vi "LVClass_Camera ctor.vi"(0 "Camera (const)":refnum<class "Camera.lvclass">, 5 "Configuration file path":path, 11 "error in (no error)":errorcluster) -> (4 "Camera (new)":refnum<class "Camera.lvclass">, 15 "error out":errorcluster)   [LabVIEW 2020, in "Camera.lvclass"]
doc: "Camera constructor.\n\n<B>CameraIn</B> : Constant Pointer to Camera object, Camera connection is automatically\n established to the device. (no neeed to use Imop_Camera_Connect)\n<B>CameraOut</B> : Constant Pointer to Camera object, Camera connection is automatically\n established to the device. (no neeed to use Imop_Camera_Connect)\n<B>config_file_path</B> : Absolute path to Haso or Camera configuration file."
uses:
  Camera.lvclass
  Handle creation.ctl
  Camera.lvclass/Camera.ctl
  CameraSet.lvclass
  Image.lvclass
  Data alignment enum.ctl
  CameraAcquisitionState.ctl
  LVClass_CameraSet Read CameraParameters.vi
  LVClass_CameraSet Read AllValueSetAndGet.vi
  LVClass_CameraSet Read AllValueGet.vi
panel:
  out "Iteration":i32
  out "State":i32
  out "path to wavekit library":path
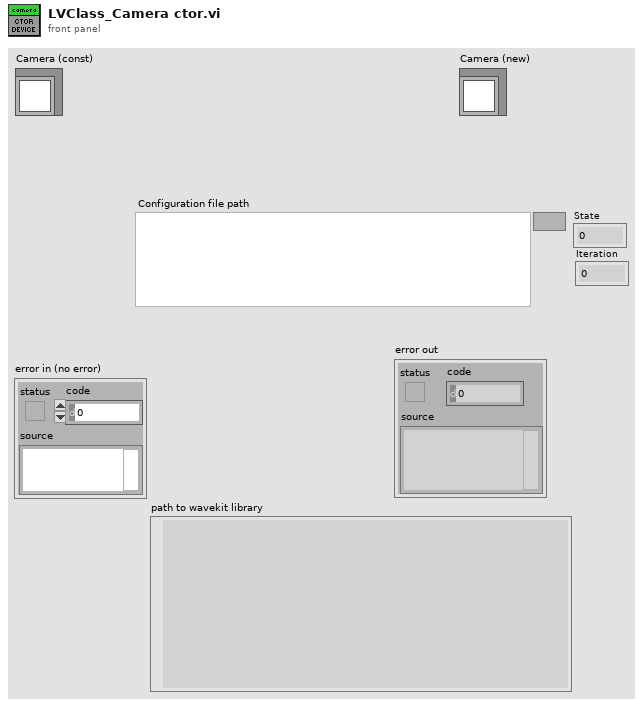
[diagram p1: front panel]
types:
  T1 = typedef "Handle creation.ctl" = enum16{"By ctor", "By write function"}
  T2 = typedef "Data alignment enum.ctl" = enum16{"8", "16", "32"}
  T3 = typedef "CameraAcquisitionState.ctl" = enum16{"Stop", "Live"}
  T4 = typedef "ParameterID.ctl" = cluster{"Name":string, "ConnectionParameter?":bool, "Type":T5, "Authorization":T6, "OnFlyAuthorization":T7, "StringValue":string, "Value":dbl, "Min":dbl, "Max":dbl, "BooleanValue":bool, "StringParameterList":string[]}
  T5 = typedef "CameraParameters_Type.ctl" = enum16{"Integer", "Real", "String", "Boolean"}
  T6 = typedef "CameraParameters_Authorization.ctl" = enum16{"Disable", "Gettable", "Settable - Gettable"}
  T7 = typedef "CameraParameters_OnFlyAuthorization.ctl" = enum16{"None", "Gettable", "Settable", "Settable - Gettable"}
  T8 = typedef "CameraParametersSetup.ctl" = cluster{"Name":string, "Type":T5, "Value":dbl, "BooleanValue":bool, "StringValue":string, "ConnectionParameter":bool}
  T9 = typedef "CameraSpecifications.ctl" = cluster{"Grabber name":string, "Camera name":string, "Camera sn":string, "Pixels_um":T10, "Maximum level":u32, "Data alignment":T2, "Is signed":bool, "Acquisition start":T11, "Acquisition length":T11, "MaxFrameRate_Hz":sgl, "Chip type":enum16{"Progressive scan", "Frame transfert"}}
  T10 = typedef "General dimensions definition.ctl" = cluster{"Size":T11, "Step":T12}
  T11 = typedef "Point2D.ctl" = cluster{"X":u32, "Y":u32}
  T12 = typedef "Point2Df.ctl" = cluster{"X":sgl, "Y":sgl}
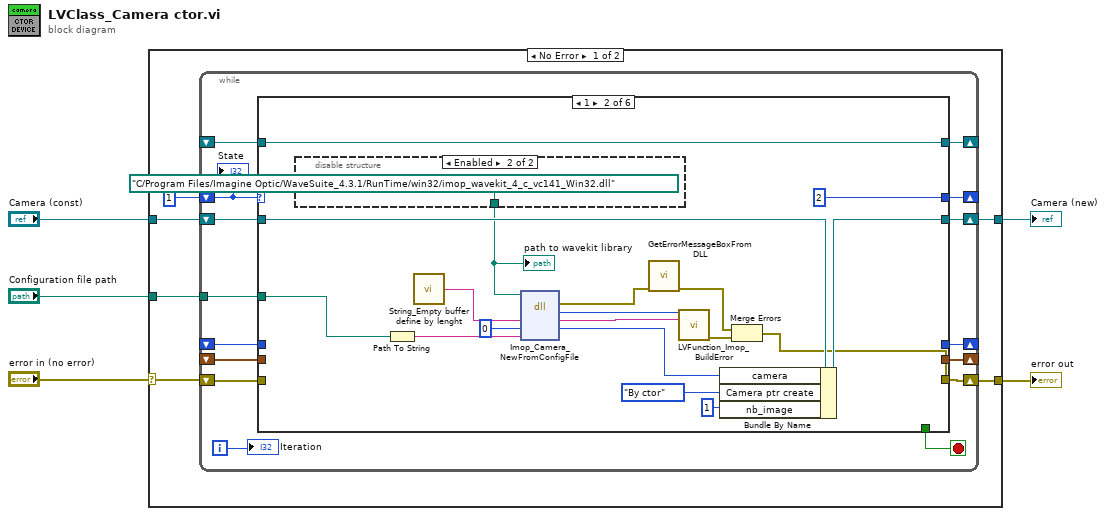
[diagram p0: block diagram]
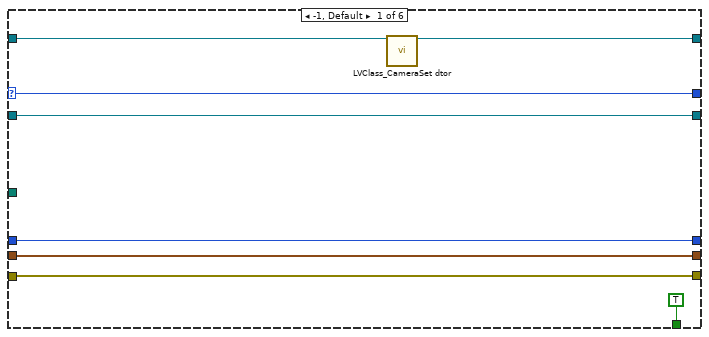
[diagram p2: hidden frame]
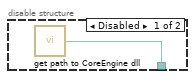
[diagram p3: hidden frame]
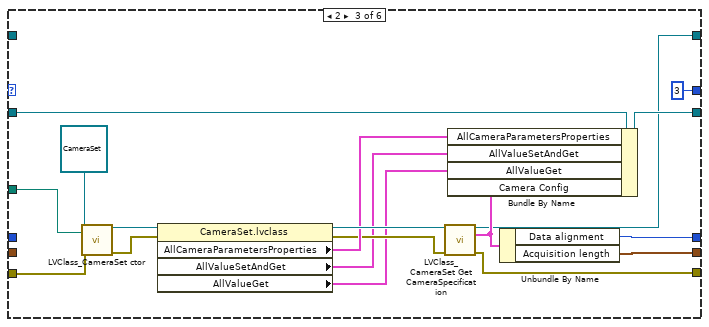
[diagram p4: hidden frame]
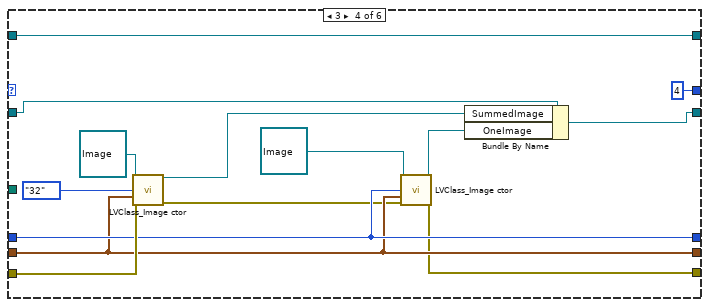
[diagram p5: hidden frame]
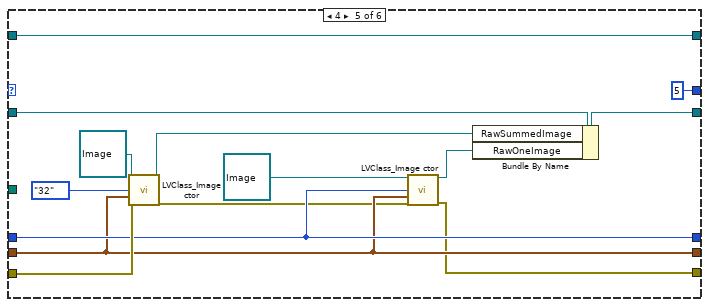
[diagram p6: hidden frame]
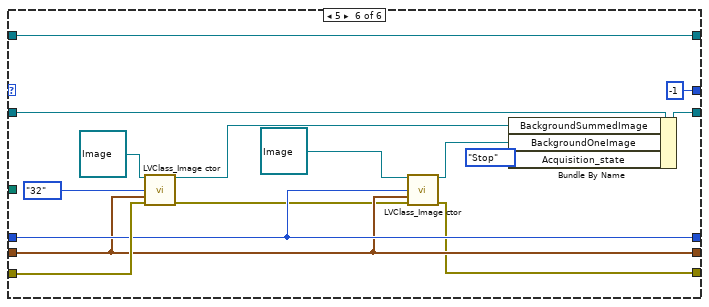
[diagram p7: hidden frame]
diagram:
  n1 = case shown="No Error" "error in (no error)" {
    selector: "error in (no error)" -> [w7 w117]
    tunnel: [w6 w117] -> w4
    tunnel: [w10 w116] -> w2
    tunnel: "Camera (const)" -> [w11 w116]
    tunnel: "Configuration file path" -> [w8 _]
    frame No Error {
      n2 = while {
        shift-right: [w24] -> _
        shift-left: 1 -> [w23]
        tunnel: w8 -> [w22]
        shift-right: [w21] -> w6
        shift-left: w7 -> [w20]
        shift-right: [w18] -> _
        shift-left: _ -> [w16]
        shift-right: [w19] -> _
        shift-left: _ -> [w17]
        shift-right: [w25] -> w10
        shift-left: w11 -> [w26]
        shift-right: [w14] -> _
        shift-left: _ -> [w13]
        i -> [w12]
        stop <- w15 stop-if-true
        n3 = case shown="1" w23 {
          selector: w23 -> [w33 _ _ _ _ _]
          tunnel: [w32 w36 w68 w76 w90 w105] -> w21
          tunnel: w26 -> [w29 w47 w65 w84 w98 w113]
          tunnel: [w29 w46 w64 w83 w97 w112] -> w25
          tunnel: [w33 2 3 4 5 -1] -> w24
          tunnel: w22 -> [_ w41 w71 _ _ _]
          tunnel: w20 -> [w32 _ w70 w85 w99 w114]
          tunnel: [w30 _ w66 w80 w94 w109] -> w19
          tunnel: [w31 _ w69 w79 w93 w108] -> w18
          tunnel: w17 -> [w30 _ _ w80 w94 w109]
          tunnel: w16 -> [w31 _ _ w79 w93 w108]
          tunnel: [TRUE _ _ _ _ _] -> w15
          tunnel: [w27 w39 w58 w74 w88 w103] -> w14
          tunnel: w13 -> [w28 w39 _ w74 w88 w103]
          frame -1, Default {
            n4 = call "LVClass_CameraSet dtor.vi"("CameraSet in"=w28) -> ("CameraSet out"=w27:refnum<class "CameraSet.lvclass">)  [unwired: 13 in, 1 out]
          }
          frame 1 {
            n5 = disable-structure shown="Enabled" {
              disable-tunnel: [w53 path "C:/Program Files/Imagine Optic/WaveSuite_4.3.1/RunTime/win32/imop_wavekit_4_c_vc141_Win32.dll" ("path to wavekit library")] -> w44
              frame Disabled {
                n6 = call "get path to CoreEngine dll.vi"() -> ("path to wavekit library"=w53:path)  [unwired: 14 in, 1 out]
              }
              frame Enabled {
              }
            }
            "path to wavekit library" <- w44
            n7 = Path To String(path=w41) -> (string=w40:string)
            n8 = call "String_Empty buffer define by lenght.vi"() -> ("Empty buffer"=w45:string)  [unwired: 1 in]
            n9 = dll-call lib="D:/soft/HASO_v3/SVN_trunk/ImOpCoreEngine4_LV2011/DLLs/c_interface_vc100.dll" fn="Imop_Camera_NewFromConfigFile"(path in=w44, "message"=w45, "objet"=0, "chemin_config"=w40) -> (error out=w43:errorcluster, "return type"=w50:i32, "message"=w49:string, "objet"=w48:i64)  [unwired: 3 in, 1 out]
            n10 = call "GetErrorMessageBoxFromDLL.vi"("error IN"=w43) -> ("error OUT"=w38:errorcluster)  [unwired: 10 in]
            n11 = call "LVFunction_Imop_BuildError.vi"("code"=w50, "String to Prepend to source (\"\")"=w49) -> ("error out"=w37:errorcluster)  [unwired: 13 in]
            n12 = Bundle By Name(cluster=w47, "camera"=w48, "Camera ptr create"=Handle_creation."By ctor" ("Haso ptr create"), "nb_image"=u32 1) -> (w46:refnum<class "Camera.lvclass">)
            n13 = Merge Errors(w38, w37) -> (w36:errorcluster)
          }
          frame 2 {
            n14 = call "LVClass_CameraSet ctor.vi"("CameraSet (const)"=refnum<class "CameraSet.lvclass"> refnum ("CameraSet.lvclass"), "Configuration file path"=w71, "error in (no error)"=w70) -> ("CameraSet (new)"=w56:refnum<class "CameraSet.lvclass">, "error out"=w55:errorcluster)  [unwired: 11 in]
            n15 = property class="CameraSet.lvclass"(reference=w56, error in=w55) -> (reference out=w63:refnum<class "CameraSet.lvclass">, error out=w61:errorcluster, "AllCameraParametersProperties"=w62:T4[], "AllValueSetAndGet"=w60:T8[], "AllValueGet"=w57:T8[])
            n16 = call "LVClass_CameraSet Get CameraSpecification.vi"("CameraSet in"=w63, "error in (no error)"=w61) -> ("CameraSet out"=w58:refnum<class "CameraSet.lvclass">, "Camera Config"=w59:T9, "error out"=w68:errorcluster)  [unwired: 11 in]
            n17 = Bundle By Name(cluster=w65, "AllCameraParametersProperties"=w62, "AllValueSetAndGet"=w60, "AllValueGet"=w57, "Camera Config"=w59) -> (w64:refnum<class "Camera.lvclass">)
            n18 = Unbundle By Name(w59) -> ("Data alignment"=w66:T2, "Acquisition length"=w69:T11)
          }
          frame 3 {
            n19 = call "LVClass_Image ctor.vi"("Image (const)"=refnum<class "Image.lvclass"> refnum ("Image in"), "Data alignment"=Data_alignment_enum."32", "Size"=w79, "error in (no error)"=w85) -> ("Image (new)"=w82:refnum<class "Image.lvclass">, "error out"=w77:errorcluster)  [unwired: 10 in]
            n20 = call "LVClass_Image ctor.vi"("Image (const)"=refnum<class "Image.lvclass"> refnum ("Image in"), "Data alignment"=w80, "Size"=w79, "error in (no error)"=w77) -> ("Image (new)"=w78:refnum<class "Image.lvclass">, "error out"=w76:errorcluster)  [unwired: 10 in]
            n21 = Bundle By Name(cluster=w84, "SummedImage"=w82, "OneImage"=w78) -> (w83:refnum<class "Camera.lvclass">)
          }
          frame 4 {
            n22 = call "LVClass_Image ctor.vi"("Image (const)"=refnum<class "Image.lvclass"> refnum ("Image in"), "Data alignment"=Data_alignment_enum."32", "Size"=w93, "error in (no error)"=w99) -> ("Image (new)"=w96:refnum<class "Image.lvclass">, "error out"=w91:errorcluster)  [unwired: 10 in]
            n23 = call "LVClass_Image ctor.vi"("Image (const)"=refnum<class "Image.lvclass"> refnum ("Image in"), "Data alignment"=w94, "Size"=w93, "error in (no error)"=w91) -> ("Image (new)"=w92:refnum<class "Image.lvclass">, "error out"=w90:errorcluster)  [unwired: 10 in]
            n24 = Bundle By Name(cluster=w98, "RawSummedImage"=w96, "RawOneImage"=w92) -> (w97:refnum<class "Camera.lvclass">)
          }
          frame 5 {
            n25 = call "LVClass_Image ctor.vi"("Image (const)"=refnum<class "Image.lvclass"> refnum ("Image in"), "Data alignment"=Data_alignment_enum."32", "Size"=w108, "error in (no error)"=w114) -> ("Image (new)"=w111:refnum<class "Image.lvclass">, "error out"=w106:errorcluster)  [unwired: 10 in]
            n26 = call "LVClass_Image ctor.vi"("Image (const)"=refnum<class "Image.lvclass"> refnum ("Image in"), "Data alignment"=w109, "Size"=w108, "error in (no error)"=w106) -> ("Image (new)"=w107:refnum<class "Image.lvclass">, "error out"=w105:errorcluster)  [unwired: 10 in]
            n27 = Bundle By Name(cluster=w113, "BackgroundSummedImage"=w111, "BackgroundOneImage"=w107, "Acquisition_state"=CameraAcquisitionState."Stop") -> (w112:refnum<class "Camera.lvclass">)
          }
        }
        "State" <- w23
        "Iteration" <- w12
      }
    }
    frame Error {
    }
  }
  "error out" <- w4
  "Camera (new)" <- w2
